vi "ATS_PrepareAcqusition.vi"(8 "error in (no error)":errorcluster, 10 "ATS Sampling":T1={"Post-trigger Samples"=2048, "Records Per Buffer"=10, "Records Count"=10}, 11 "Handle in":u32) -> (0 "error out":errorcluster, 2 "Array":u16[](array[numeric]), 3 "Handle out":u32)   [LabVIEW 2016]
uses:
  CTL/ATS_Sampling.ctl
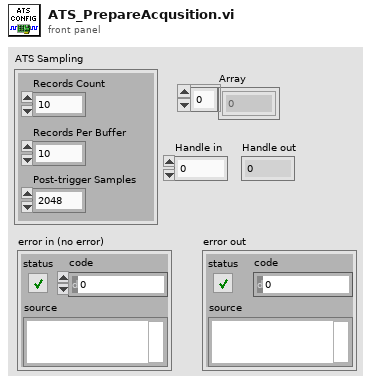
[diagram p1: front panel]
types:
  T1 = typedef "ATS_Sampling.ctl" = cluster{"Post-trigger Samples":u32, "Records Per Buffer":u32, "Records Count":u32}
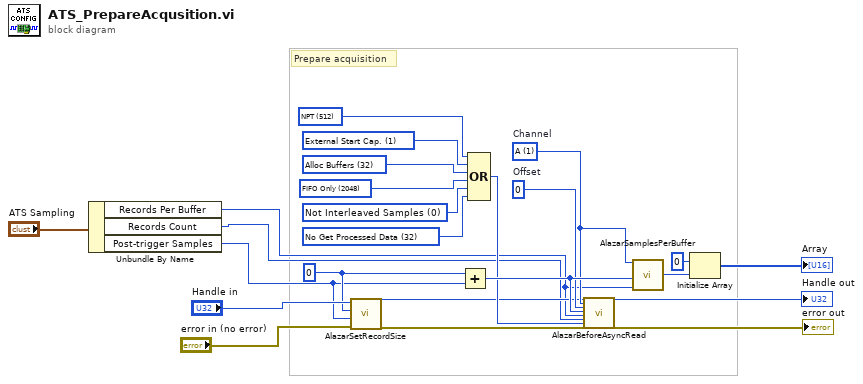
[diagram p0: block diagram]
diagram:
  w15 = u32 0  # Offset
  w23 = u32 1 items=["A"=1, "B"=2, "A + B"=3, "C"=4, "A + C"=5, "A + B"=6, "D"=8, "A + D"=9, "B + D"=10, "C + D"=12, "A + B + C + D"=15]  # Channel
  w11 = u32 0 ("Pre-trigger Samples")
  w5 = u32 32 items=["No Get Processed Data"=32, "Get Processed Data"=8192]
  w6 = u32 0 items=["Not Interleaved Samples"=0, "Interleave Samples"=4096]
  w10 = u32 2048 items=["No FIFO Only"=0, "FIFO Only"=2048]
  w7 = u32 32 items=["Alloc Buffers"=32]
  w8 = u32 1 items=["Internal Start Cap.", "External Start Cap."]
  w9 = u32 512 items=["Traditional"=0, "NPT"=512, "Continuous"=256, "Triggered Streaming"=1024]
  # "Prepare acquisition"
  n1 = Unbundle By Name("ATS Sampling") -> ("Records Per Buffer"=w1:u32, "Records Count"=w3:u32, "Post-trigger Samples"=w2:u32)
  n2 = call "AlazarSetRecordSize.vi"("error in (no error)"="error in (no error)", "Post-trigger Samples"=w2, "Pre-trigger Samples"=w11, "Handle"="Handle in") -> ("error out"=w13:errorcluster, "Handle"=w12:u32)  [unwired: 1 out]
  n3 = Add(x=w11, y=w2) -> (x+y=w24:u32)
  n4 = Compound Arithmetic op=OR(w9, w8, w7, w10, w6, w5) -> (w14:u32)
  n5 = call "AlazarBeforeAsyncRead.vi"("Handle"=w12, "Channel"=w23, "Offset"=w15, "Length"=w24, "Records Per Buffer"=w1, "Records Count"=w3, "cFlags"=w14, "error in (no error)"=w13) -> ("Handle"=→"Handle out":u32, "error out"=→"error out":errorcluster)  [unwired: 17 in, 1 out]
  n6 = call "AlazarSamplesPerBuffer.vi"("Records Per Buffer"=w1, "Samples Per Record"=w24, "Channel Mask"=w23) -> ("Samples Per Buffer"=w22:u32)  [unwired: 1 in]
  n7 = Initialize Array(u16 0, w22) -> (→"Array":u16[])
